vi "Wrist Angle.vi"(9 "Belt Reduction":dbl=2.75, 10 "Ticks/Rev":dbl=4096.0, 11 "Ticks (from vertical)":dbl) -> (2 "Angle (Radians)":dbl, 3 "Angle (degrees from vertical)":dbl)   [LabVIEW 2018]
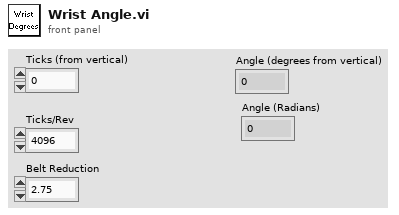
[diagram p1: front panel]
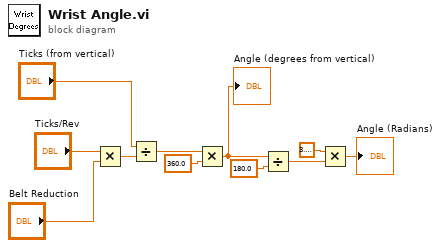
[diagram p0: block diagram]
diagram:
  n1 = Multiply(x="Ticks/Rev", y="Belt Reduction") -> (x*y=w9:dbl)
  n2 = Divide(x="Ticks (from vertical)", y=w9) -> (x/y=w7:dbl)
  n3 = Multiply(x=w7, y=360.0) -> (x*y=w4:dbl)
  "Angle (degrees from vertical)" <- w4
  n4 = Divide(x=w4, y=180.0) -> (x/y=w3:dbl)
  n5 = Multiply(x=3.141592653589793, y=w3) -> (x*y=→"Angle (Radians)":dbl)
